vi "Eth Status Manager Close.vi"(8 "error in":errorcluster, 11 "Status Reference":T1) -> (0 "error out":errorcluster)   [LabVIEW 2021, in "Eth Status.lvlib"]
uses:
  Eth Status.lvlib
  Ctl/Status.ctl
  MB_TCP2/MB_TCP_State.ctl
  MB_TCP2/MB_TCP.lvclass
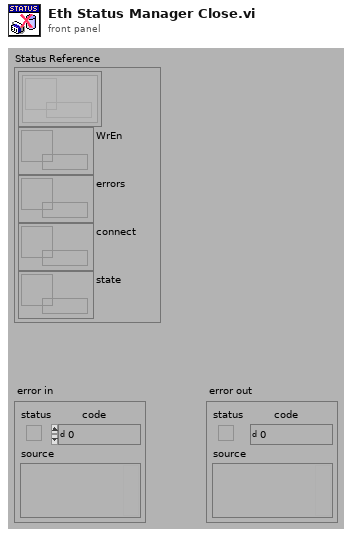
[diagram p1: front panel]
types:
  T1 = typedef "Eth Status.lvlib/Status.ctl" = cluster{"Set_states":refnum<queue>[], "WrEn":refnum<data-value>, "errors":refnum<data-value>, "connect":refnum<data-value>, "state":refnum<data-value>}
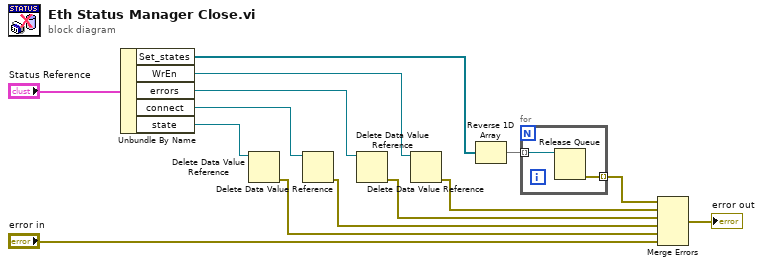
[diagram p0: block diagram]
diagram:
  n1 = Unbundle By Name("Status Reference") -> ("Set_states"=w2:refnum<queue>[], "WrEn"=w14:refnum<data-value>, "errors"=w13:refnum<data-value>, "connect"=w9:refnum<data-value>, "state"=w7:refnum<data-value>)
  n2 = Delete Data Value Reference(data value reference=w7) -> (error out=w6:errorcluster)  [unwired: 1 in, 1 out]
  n3 = Delete Data Value Reference(data value reference=w9) -> (error out=w8:errorcluster)  [unwired: 1 in, 1 out]
  n4 = Delete Data Value Reference(data value reference=w13) -> (error out=w11:errorcluster)  [unwired: 1 in, 1 out]
  n5 = Delete Data Value Reference(data value reference=w14) -> (error out=w12:errorcluster)  [unwired: 1 in, 1 out]
  n6 = Reverse 1D Array(array=w2) -> (reversed array=w3:refnum<queue>[])
  n7 = for {
    tunnel: w3 -> [w16] mode=indexing
    tunnel: [w15] -> w1 mode=indexing
    n8 = Release Queue(queue=w16) -> (error out=w15:errorcluster)  [unwired: 2 in, 2 out]
  }
  n9 = Merge Errors(w1, w12, w11, w8, w6, "error in") -> (→"error out":errorcluster)
